vi "DCMotor_GetRomiBuiltIn.vi"(11 "Num Motors":i32=1) -> (3 "DCMOTOR":T1 {"Jr_KgM2" format="%13.5p"; "L_H" format="%13.5p"; "Kt_NMPerAmp" format="%13.5p"; "KvINV_RadPerSecPerVolt" format="%13.5p"; "R_Ohms" format="%13.5p"; "FreeSpeed_RadPerSec" format="%13.5p"; "FreeCurrent_Amps" format="%13.5p"; "StallCurrent_Amps" format="%13.5p"; "StallTorque_NM" format="%13.5p"; "nominalVoltage_Volts" format="%13.5p"})   [LabVIEW 2019, in "Trajectory_Library.lvlib"]
doc: "Creates a new DC MOTOR data cluster with the specified values. for a set of Romi Built In motors. \n\nInputs: \n - Num Motors -- The number of motors used together in this sytem driving the same load.\n\nOutputs:\n - DCMOTOR -- Cluster containing the motor modeling constants for this set of motors."
uses:
  Trajectory_Library.lvlib
  TypeDef/DCMOTOR.CTL
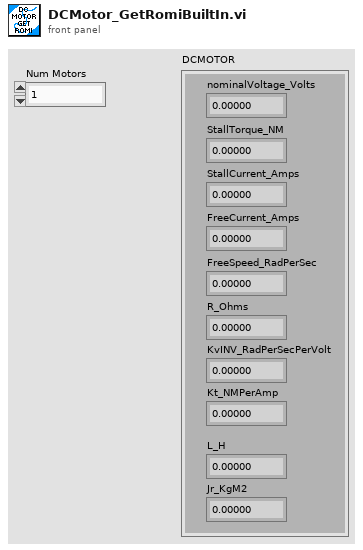
[diagram p1: front panel]
types:
  T1 = typedef "Trajectory_Library.lvlib/DCMOTOR.CTL" = cluster{"nominalVoltage_Volts":dbl, "StallTorque_NM":dbl, "StallCurrent_Amps":dbl, "FreeCurrent_Amps":dbl, "FreeSpeed_RadPerSec":dbl, "R_Ohms":dbl, "KvINV_RadPerSecPerVolt":dbl, "Kt_NMPerAmp":dbl, "L_H":dbl, "Jr_KgM2":dbl}
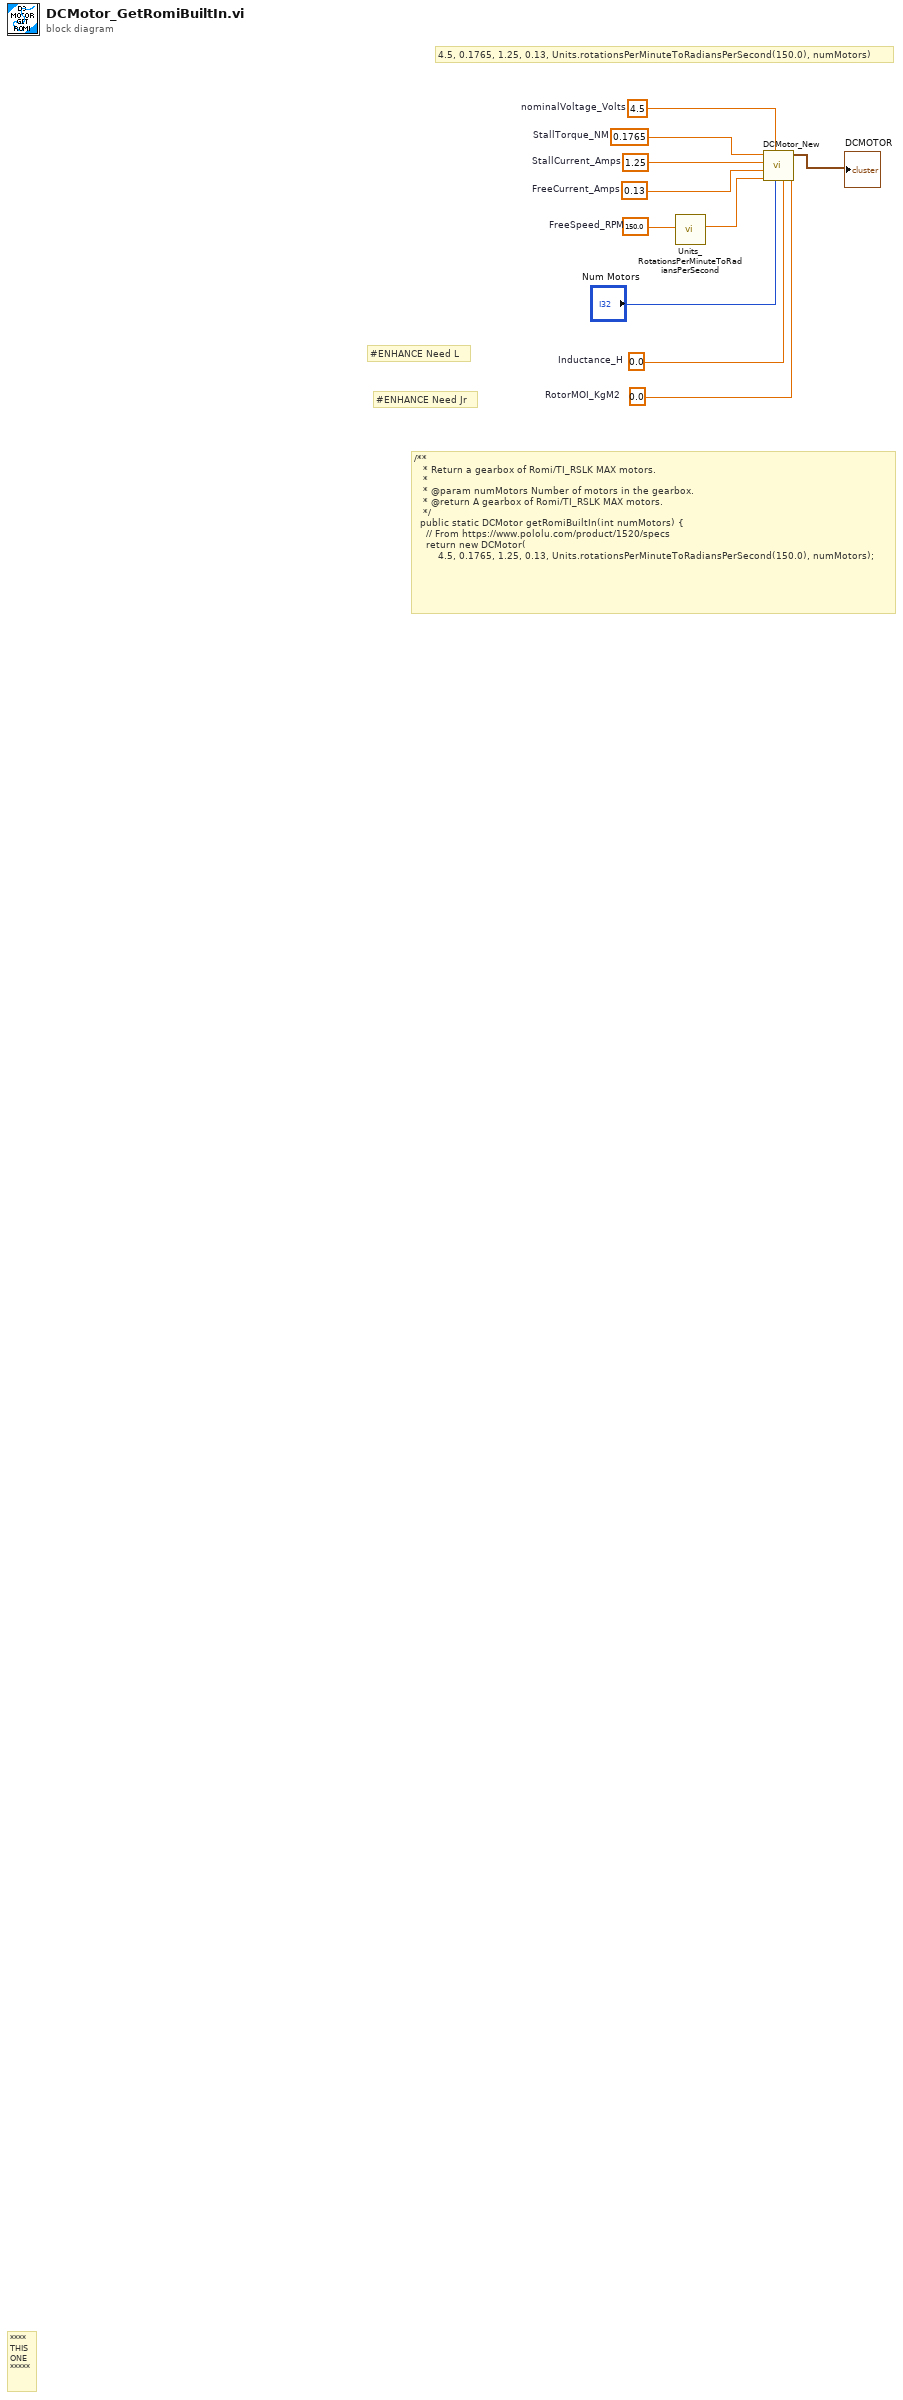
[diagram p0: block diagram]
diagram:
  w2 = 0.0  # RotorMOI_KgM2
  w1 = 0.0  # Inductance_H
  w4 = 150.0  # FreeSpeed_RPM
  w5 = 0.13  # FreeCurrent_Amps
  w6 = 1.25  # StallCurrent_Amps
  w7 = 0.1765  # StallTorque_NM
  w8 = 4.5  # nominalVoltage_Volts
  # "#ENHANCE Need Jr"
  # "#ENHANCE Need L"
  # "4.5, 0.1765, 1.25, 0.13, Units.rotationsPerMinuteToRadiansPerSecond(150.0), numMotors)"
  # "/**\n   * Return a gearbox of Romi/TI_RSLK MAX motors.\n   *\n   * @param numMotors Number of motors in the gearbox.\n   * @return A gearbox of Romi/TI_RSLK MAX motors.\n   */\n  public static DCMotor getRomiBuiltIn(int numMotors) {\n    // From https://www.pololu.com/product/1520/specs\n    return new DCMotor(\n        4.5, 0.1765, 1.25, 0.13, Units.rotationsPerMinuteToRadiansPerSecond(150.0), numMotors);"
  # "****\nTHIS\nONE\n*****"
  n1 = call "Units_RotationsPerMinuteToRadiansPerSecond.vi"("RotationsPerMinute"=w4) -> ("RadiansPerSecond"=w3:dbl)  [unwired: 10 in]
  n2 = call "DCMotor_New.vi"("RotorMOI_KgM2"=w2, "Inductance_H"=w1, "Num Motors"="Num Motors", "nominalVoltage_Volts"=w8, "FreeSpeed_RadPerSec"=w3, "FreeCurrent_Amps"=w5, "StallCurrent_Amps"=w6, "StallTorque_NM"=w7) -> ("DCMOTOR"=→"DCMOTOR":T1)  [unwired: 3 in]
